vi "Prime_timer.vi"() -> ()   [LabVIEW 2010]
uses:
  Globals/Trav_pos_global.vi
panel:
  in  "Setup filename":path
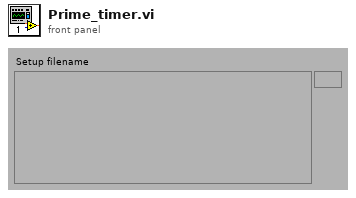
[diagram p1: front panel]
types:
  T1 = typedef "Traverse_cluster.ctl" = cluster{"Start X":dbl, "Start Y":dbl, "Start Z":dbl, "End X":dbl, "End Y":dbl, "End Z":dbl, "No. of pts.":i32, "Spacing":T2, "Filename":path, "Tunnel Speed":dbl, "Averaging time (min)":dbl, "Extra Commands":string, "Specific Arguments":string, "Emission Rate (l/min)":dbl, "Trace Gas Concentration (%)":dbl, "Density Ratio":string, "Comments":string, "Row No":i32, "Row Type Selector":T3, "Completion time":string, "Row Duration (mins)":dbl, "No. of Valid pts.":i32, "Meas Setup File":string}
  T2 = typedef "Spacing.ctl" = enum16{"Linear", "Log", "Gauss", "Specified", "N/A"}
  T3 = typedef "Multi_run_mode.ctl" = enum16{"Move Traverse Only", "Set Tunnel Speed Only", "Set Source Only", "Set Measurement Conditions", "Single Measurement", "Vertical Profile", "Lateral Profile", "Longitudinal Profile", "Explore Volume", "Multi-Axis Profile", "Auto Calibrate", "Meas Fast FID Bkgnd", "Check Beam Power", "Scanning Valve Measurement", "Run VI Named:", "Set ADAM Ch", "Wait (minutes)", "Send Message", "Synchronize With:", "Fall Back to this Row", "Turn Off Row Repeating", "Blank Row"}
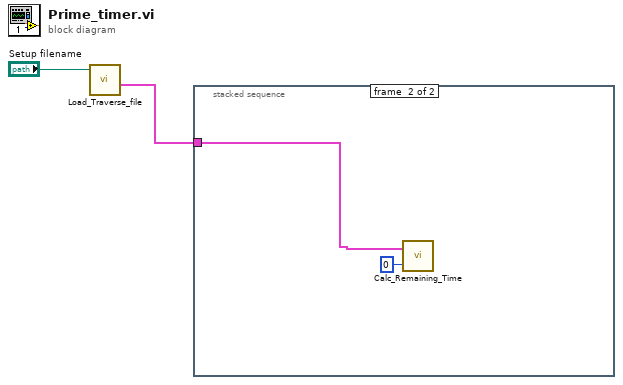
[diagram p0: block diagram]
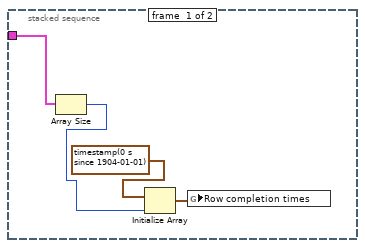
[diagram p2: hidden frame]
diagram:
  n1 = call "Load_Traverse_file.vi"("Setup filename"="Setup filename") -> ("Table"=w1:T1[])  [unwired: 2 in, 3 out]
  n2 = stacked-sequence {
    tunnel: w1 -> [w4 w8]
    frame #0 {
      n3 = Array Size(array=w4) -> (size(s)=w3:i32)
      n4 = Initialize Array(timestamp(0 s since 1904-01-01) ("seconds since 1Jan1904"), w3) -> (w5:timestamp[])
      n5 = global write "Trav_pos_global.vi" "Row completion times"(w5) -> ()
    }
    frame #1 {
      n6 = call "Calc_Remaining_Time.vi"("Currently on Row"=0, "Table In"=w8) -> ()  [unwired: 2 out]
    }
  }
